vi "Setup UI.vi"(8 "error in (no error)":errorcluster, 10 "Set UI to input? (F)":bool, 11 "Wavelength in":refnum<class "Wavelength.lvclass">) -> (0 "error out":errorcluster, 3 "Wavelength out":refnum<class "Wavelength.lvclass">)   [LabVIEW 2009, in "Wavelength.lvclass"]
uses:
  Wavelength.lvclass
  Wavelength.lvclass/Wavelength.ctl
panel:
  in  "Optimize":enum32{"Slits", "Step Size"}(radio)=enum."Step Size"
  in  "Step size":dbl[unit] caption="Recommended step size\n(must enter above too)"
  in  "Lateral Exit":dbl[unit]
  in  "Axial Entrance":dbl[unit]
  # "Wavelength Scan Setup"
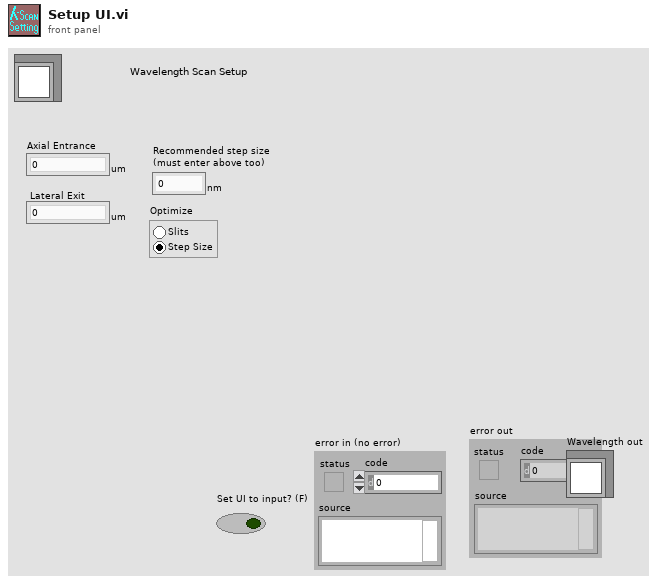
[diagram p1: front panel]
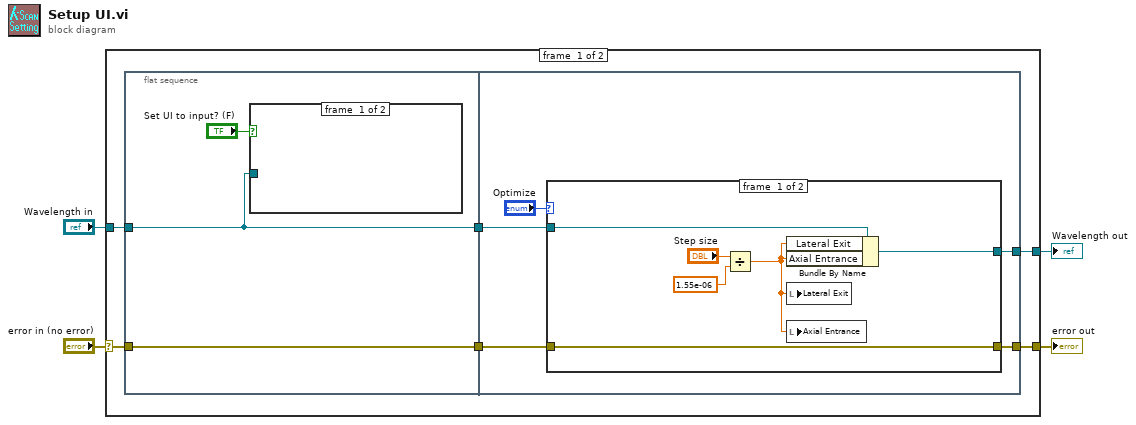
[diagram p0: block diagram]
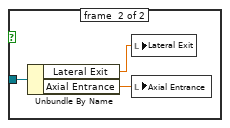
[diagram p2: hidden frame]
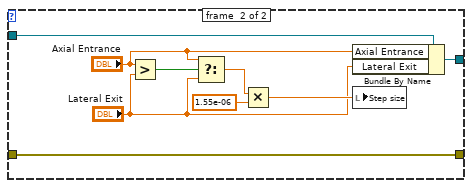
[diagram p3: hidden frame]
diagram:
  n1 = case shown="No Error" "error in (no error)" {
    selector: "error in (no error)" -> [w9 w37]
    tunnel: [w10 w37] -> w3
    tunnel: "Wavelength in" -> [w8 w38]
    tunnel: [w7 w38] -> w1
    frame #0 {
      n2 = flat-sequence {
        tunnel: w8 -> [w11]
        tunnel: w9 -> [w13]
        tunnel: [w13] -> w6
        tunnel: [w11] -> w5
        tunnel: w6 -> [w19]
        tunnel: w5 -> [w18]
        tunnel: [w20] -> w10
        tunnel: [w17] -> w7
        frame #0 {
          n3 = case shown="True" "Set UI to input? (F)" {
            tunnel: w11 -> [_ w16]
            frame #0 {
            }
            frame #1 {
              n4 = Unbundle By Name(w16) -> ("Lateral Exit"=w15:dbl[unit], "Axial Entrance"=w14:dbl[unit])
              n5 = local write "Lateral Exit"(w15) -> ()
              n6 = local write "Axial Entrance"(w14) -> ()
            }
          }
        }
        frame #1 {
          n7 = case shown="\"Step Size\"" "Optimize" {
            tunnel: [w25 w32] -> w20
            tunnel: w19 -> [w25 w32]
            tunnel: w18 -> [w24 w33]
            tunnel: [w23 w30] -> w17
            frame #0 {
              n8 = Divide(x="Step size", y=1.55e-06) -> (x/y=w22:dbl[unit])
              n9 = Bundle By Name(cluster=w24, "Lateral Exit"=w22, "Axial Entrance"=w22) -> (w23:refnum<class "Wavelength.lvclass">)
              n10 = local write "Lateral Exit"(w22) -> ()
              n11 = local write "Axial Entrance"(w22) -> ()
            }
            frame #1 {
              n12 = Greater?(x="Axial Entrance", y="Lateral Exit") -> (0:w35:bool)
              n13 = Select(t="Axial Entrance", s=w35, f="Lateral Exit") -> (s? t:f=w34:dbl[unit])
              n14 = Multiply(x=w34, y=1.55e-06) -> (x*y=w31:dbl[unit])
              n15 = Bundle By Name(cluster=w33, "Axial Entrance"="Axial Entrance", "Lateral Exit"="Lateral Exit") -> (w30:refnum<class "Wavelength.lvclass">)
              n16 = local write "Step size"(w31) -> ()
            }
          }
        }
      }
    }
    frame #1 {
    }
  }
  "error out" <- w3
  "Wavelength out" <- w1
